vi "testbaby (SubVI).vi"(5 "- move":bool, 6 "Axis Speeds":T2={"X [mm/s]"=10.0, "Y [mm/s]"=10.0, "Z [mm/s]"=10.0}, 7 "+ move":bool, 9 "Axis name":string(combo), 10 "Jog step size":T1={"X [mm]"=0.001, "Y [mm]"=0.001, "Z [mm]"=0.001}) -> (3 "Current stage position [mm]":cluster{"X":dbl, "Y":dbl, "Z":dbl})   [LabVIEW 2016]
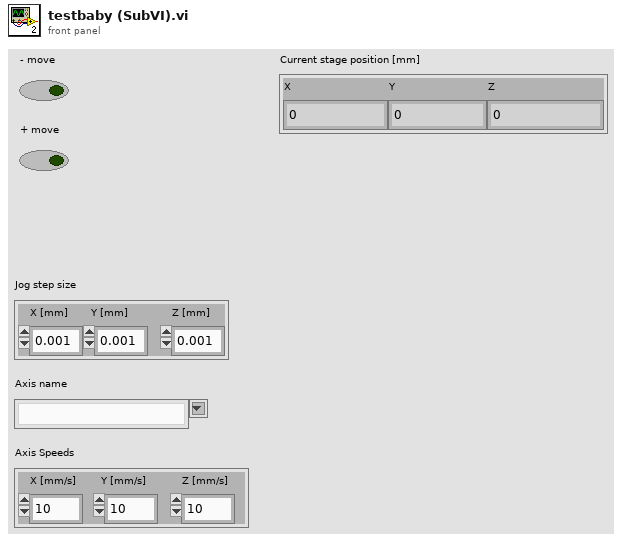
[diagram p1: front panel]
types:
  T1 = cluster{"X [mm]":dbl, "Y [mm]":dbl, "Z [mm]":dbl}
  T2 = cluster{"X [mm/s]":dbl, "Y [mm/s]":dbl, "Z [mm/s]":dbl}
  T3 = cluster{"X Position Feedback":dbl, "Y Position Feedback":dbl, "Z Position Feedback":dbl}
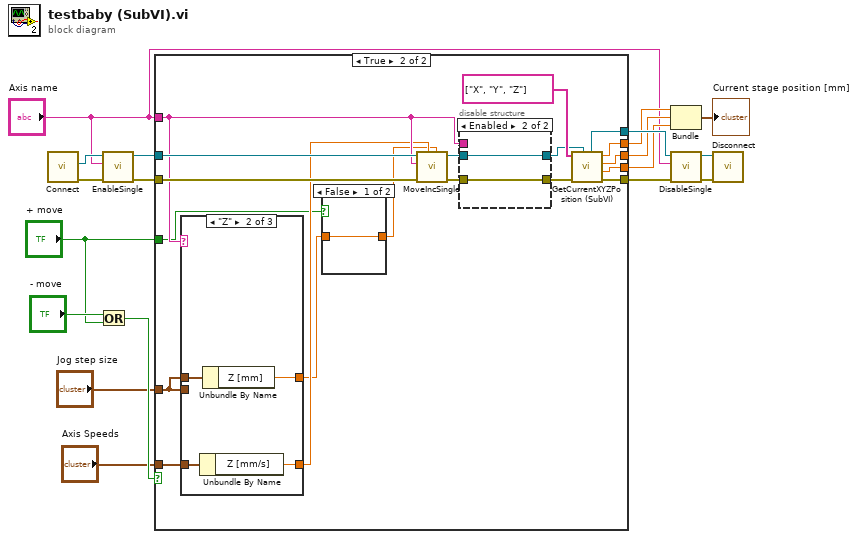
[diagram p0: block diagram]
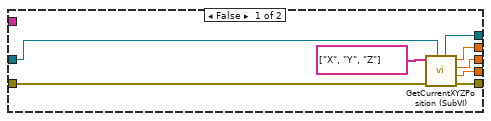
[diagram p2: hidden frame]
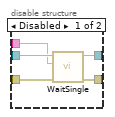
[diagram p3: hidden frame]
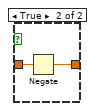
[diagram p4: hidden frame]
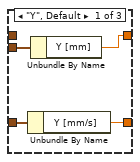
[diagram p5: hidden frame]
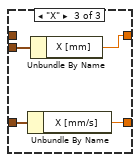
[diagram p6: hidden frame]
diagram:
  n1 = call "Connect.vi"() -> ("error out"=w17:errorcluster, "controller"=w18:refnum<k24>)  [unwired: 10 in]
  n2 = Or(x="- move", y="+ move") -> (x .or. y?=w15:bool)
  n3 = call "EnableSingle.vi"("error in (no error)"=w17, "axis name"="Axis name", "controller in"=w18) -> ("error out"=w9:errorcluster, "controller out"=w10:refnum<k24>)  [unwired: 7 in]
  n4 = case shown="True" w15 {
    tunnel: [w24 w43] -> w14
    tunnel: [w20 w42] -> w12
    tunnel: w10 -> [w25 w39]
    tunnel: "Axis name" -> [_ w36]
    tunnel: w9 -> [w19 w38]
    tunnel: "Jog step size" -> [_ w33]
    tunnel: "Axis Speeds" -> [_ w34]
    tunnel: [w23 w32] -> w6
    tunnel: [w22 w31] -> w5
    tunnel: [w21 w30] -> w4
    tunnel: "+ move" -> [_ w27]
    frame False {
      n5 = call "GetCurrentXYZPosition (SubVI).vi"(".NET Refnum in - Device"=w25, "error in (no error)"=w19, "Axes Names"=string[] ["X", "Y", "Z"]) -> ("error out"=w20:errorcluster, "Z Position Feedback"=w21:dbl, "Y Position Feedback"=w22:dbl, "X Position Feedback"=w23:dbl, ".NET Refnum out  - Device"=w24:refnum<k24>)  [unwired: 3 in]
    }
    frame True {
      n6 = case shown="\"Z\"" w36 {
        tunnel: w33 -> [w57 _ w67]
        tunnel: [w56 w60 w66] -> w29
        tunnel: [w59 w62 w65] -> w35
        tunnel: w34 -> [w58 w63 w64]
        tunnel: w33 -> [_ w61 _]
        frame "Y", Default {
          n7 = Unbundle By Name(w58) -> ("Y [mm/s]"=w59:dbl)
          n8 = Unbundle By Name(w57) -> ("Y [mm]"=w56:dbl)
        }
        frame "Z" {
          n9 = Unbundle By Name(w63) -> ("Z [mm/s]"=w62:dbl)
          n10 = Unbundle By Name(w61) -> ("Z [mm]"=w60:dbl)
        }
        frame "X" {
          n11 = Unbundle By Name(w64) -> ("X [mm/s]"=w65:dbl)
          n12 = Unbundle By Name(w67) -> ("X [mm]"=w66:dbl)
        }
      }
      n13 = case shown="False" w27 {
        tunnel: w29 -> [w53 w55]
        tunnel: [w53 w54] -> w28
        frame False {
        }
        frame True {
          n14 = Negate(x=w55) -> (-x=w54:dbl)
        }
      }
      n15 = call "MoveIncSingle.vi"("distance"=w28, "speed"=w35, "error in (no error)"=w38, "axis name"=w36, "controller in"=w39) -> ("error out"=w37:errorcluster, "controller out"=w40:refnum<k24>)  [unwired: 5 in]
      n16 = disable-structure shown="Enabled" {
        disable-tunnel: [w50 w52] -> w44
        disable-tunnel: [w49 w51] -> w41
        disable-tunnel: w40 -> [w48 w52]
        disable-tunnel: w37 -> [w47 w51]
        disable-tunnel: w36 -> [w46 _]
        frame Disabled {
          n17 = call "WaitSingle.vi"("error in (no error)"=w47, "axis name"=w46, "controller in"=w48) -> ("error out"=w49:errorcluster, "controller out"=w50:refnum<k24>)  [unwired: 6 in, 1 out]
        }
        frame Enabled {
        }
      }
      n18 = call "GetCurrentXYZPosition (SubVI).vi"(".NET Refnum in - Device"=w44, "error in (no error)"=w41, "Axes Names"=string[] ["X", "Y", "Z"]) -> ("error out"=w42:errorcluster, "Z Position Feedback"=w30:dbl, "Y Position Feedback"=w31:dbl, "X Position Feedback"=w32:dbl, ".NET Refnum out  - Device"=w43:refnum<k24>)  [unwired: 3 in]
    }
  }
  n19 = Bundle("X Position Feedback"=w6, "Y Position Feedback"=w5, "Z Position Feedback"=w4) -> (→"Current stage position [mm]":T3)  [unwired: 1 in]
  n20 = call "DisableSingle.vi"("error in (no error)"=w12, "axis name"="Axis name", "controller in"=w14) -> ("error out"=w11:errorcluster, "controller out"=w13:refnum<k24>)  [unwired: 7 in]
  n21 = call "Disconnect.vi"("error in (no error)"=w11, "controller"=w13) -> ()  [unwired: 9 in, 1 out]
